vi "Substitute Actor.vi"(10 "Substitute Actor in":refnum<class "Actor.lvclass">, 11 "Current EL-Go To Height":refnum<class "EL-Go To Height.lvclass">) -> (0 "error out":errorcluster, 2 "Substitute Actor out":refnum<class "Actor.lvclass">)   [LabVIEW 2014, in "Elevator.lvlib" / "EL-Go To Height.lvlib" / "EL-Go To Height.lvclass"]
doc: "(<B>Filename</B>: Actor Framework.lvlib:Actor.lvclass:Substitute Actor.vi)\n\nThis method copies information from the <b>Current Actor</b> to the <b>Substitute Actor</b>, including the to-self and the to-caller queue references. The purpose of this function is to allow an actor to define a method that replaces itself with another actor, useful for implementing a State Pattern Actor. Child classes should override this method to copy any additional fields that they need from the current to the substitute.\n\nThis method may return error code 678010: Illegal substitution. Overrides of this method may choose to return this error if the new actor is not one that is an appropriate substitute for the current actor, for whatever standards of \"appropriate\" are chosen for the current actor. If returning an error, override VIs should return the unmodified <b>Current Actor</b> as <b>Substitute Actor out</b>."
uses:
  EL-Go To Height.lvclass
  <vilib>/ActorFramework/Actor/Actor.lvclass
  EL-Go To Height.lvclass/EL-Go To Height.ctl
  Robot Actor Framework/Command Actor/Command Actor Class/Command Actor.lvclass
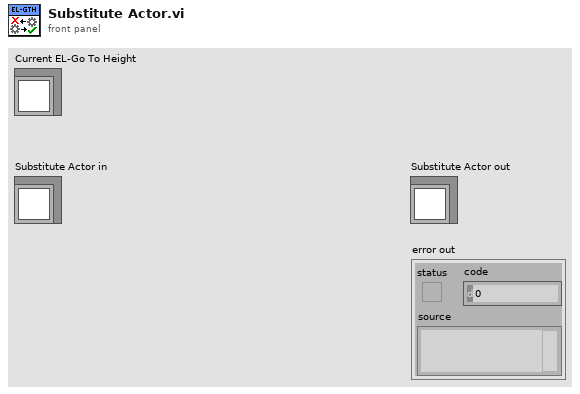
[diagram p1: front panel]
types:
  T1 = typedef "Elevator.lvlib/EL-Go To Height.lvlib/EL-Go To Height.lvclass/Parameters.ctl" = cluster{"Target Height":dbl, "Elevator State Loop (ms)":u32, "Up Rate (Percentage)":dbl, "Down Rate (Percentage)":dbl}
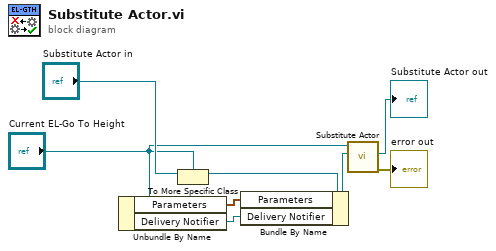
[diagram p0: block diagram]
diagram:
  n1 = Unbundle By Name("Current EL-Go To Height") -> ("Parameters"=w2:T1, "Delivery Notifier"=w1:refnum<notifier>)
  n2 = To More Specific Class(target class="Current EL-Go To Height", reference="Substitute Actor in") -> (specific class reference=w5:refnum<class "EL-Go To Height.lvclass">)  [unwired: 1 in, 1 out]
  n3 = Bundle By Name(cluster=w5, "Parameters"=w2, "Delivery Notifier"=w1) -> (w3:refnum<class "EL-Go To Height.lvclass">)
  n4 = call-parent "Substitute Actor.vi"("Substitute Actor in"=w3, "Current Command Actor"="Current EL-Go To Height") -> ("error out"=→"error out":errorcluster, "Substitute Actor out"=→"Substitute Actor out":refnum<class "Actor.lvclass">)  [unwired: 8 in]
